vi "Reactor Coolant Pump Motor Speed.vi"(0 "SI600.lvclass in":refnum<class "SI600.lvclass">, 1 "3 JEB CS951 XQ01":dbl, 2 "3 JEB CS952 XQ01":dbl, 3 "3 JEB CS953 XQ01":dbl, 4 "3 JEB CS954 XQ01":dbl, 5 "error in":errorcluster) -> (14 "SI600.lvclass out":refnum<class "SI600.lvclass">, 15 "RCP20 Speed":dbl, 16 "Speed Calculations":T2, 17 "Speed per Loop":T1, 19 "error IO":errorcluster)   [LabVIEW 2022 SP3, in "SI600.lvclass"]
uses:
  SI600.lvclass
  SI600.lvclass/SI600.ctl
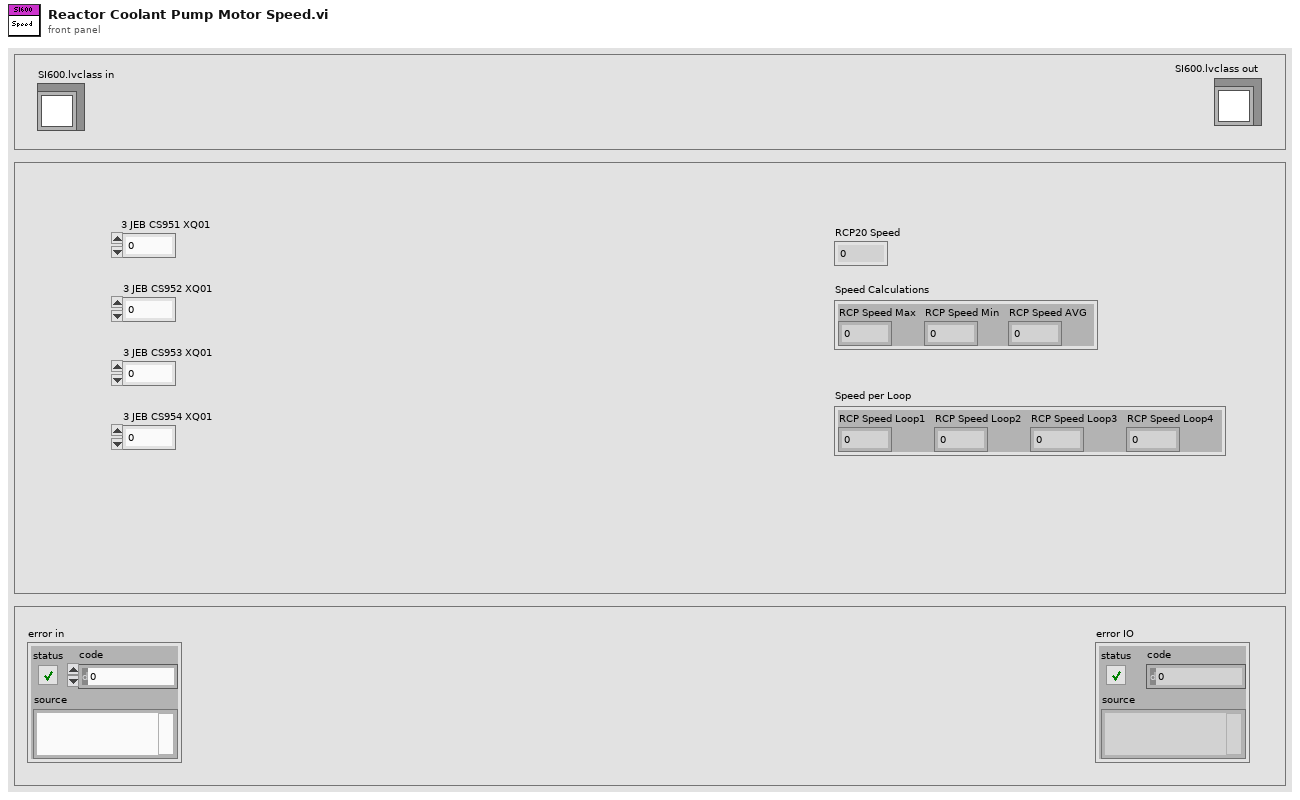
[diagram p1: front panel]
types:
  T1 = cluster{"RCP Speed Loop1":dbl, "RCP Speed Loop2":dbl, "RCP Speed Loop3":dbl, "RCP Speed Loop4":dbl}
  T2 = cluster{"RCP Speed Max":dbl, "RCP Speed Min":dbl, "RCP Speed AVG":dbl}
  T3 = cluster{"3 JEB CS951 ":dbl, "3 JEB CS952":dbl, "3 JEB CS953":dbl, "3 JEB CS954":dbl}
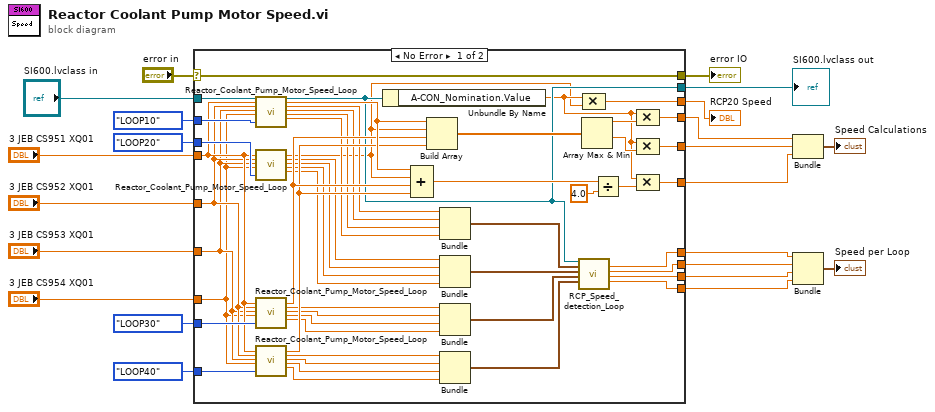
[diagram p0: block diagram]
diagram:
  n1 = case shown="No Error" "error in" {
    selector: "error in" -> [w27 w73]
    tunnel: enum16{"LOOP10", "LOOP20", "LOOP30", "LOOP40"}."LOOP10" ("Loop") -> [w69 _]
    tunnel: enum16{"LOOP10", "LOOP20", "LOOP30", "LOOP40"}."LOOP20" ("Loop") -> [w68 _]
    tunnel: enum16{"LOOP10", "LOOP20", "LOOP30", "LOOP40"}."LOOP30" ("Loop") -> [w72 _]
    tunnel: enum16{"LOOP10", "LOOP20", "LOOP30", "LOOP40"}."LOOP40" ("Loop") -> [w71 _]
    tunnel: "SI600.lvclass in" -> [w70 w74]
    tunnel: [w37 w74] -> w16
    tunnel: [w41 _] -> w9
    tunnel: [w40 _] -> w8
    tunnel: [w39 _] -> w7
    tunnel: [w38 _] -> w6
    tunnel: [w35 _] -> w12
    tunnel: [w33 _] -> w13
    tunnel: [w31 _] -> w11
    tunnel: [w28 _] -> w15
    tunnel: [w27 w73] -> w14
    tunnel: "3 JEB CS951 XQ01" -> [w26 _]
    tunnel: "3 JEB CS952 XQ01" -> [w25 _]
    tunnel: "3 JEB CS953 XQ01" -> [w24 _]
    tunnel: "3 JEB CS954 XQ01" -> [w23 _]
    frame No Error {
      n2 = call "Reactor_Coolant_Pump_Motor_Speed_Loop.vi"("SI600.lvclass in"=w70, "3 JEB CS951 XQ01"=w26, "3 JEB CS952 XQ01"=w25, "3 JEB CS953 XQ01"=w24, "3 JEB CS954 XQ01"=w23, "Loop"=w69) -> ("SI600.lvclass out"=w37:refnum<class "SI600.lvclass">, "RCP speed Loop Output"=w66:dbl, "3 JEB CS951"=w61:dbl, "3 JEB CS952"=w60:dbl, "3 JEB CS953"=w59:dbl, "3 JEB CS954"=w58:dbl)  [unwired: 15 in, 1 out]
      n3 = call "Reactor_Coolant_Pump_Motor_Speed_Loop.vi"("3 JEB CS951 XQ01"=w26, "3 JEB CS952 XQ01"=w25, "3 JEB CS953 XQ01"=w24, "3 JEB CS954 XQ01"=w23, "Loop"=w68) -> ("RCP speed Loop Output"=w29:dbl, "3 JEB CS951"=w56:dbl, "3 JEB CS952"=w55:dbl, "3 JEB CS953"=w54:dbl, "3 JEB CS954"=w53:dbl)  [unwired: 16 in, 2 out]
      n4 = call "Reactor_Coolant_Pump_Motor_Speed_Loop.vi"("3 JEB CS951 XQ01"=w26, "3 JEB CS952 XQ01"=w25, "3 JEB CS953 XQ01"=w24, "3 JEB CS954 XQ01"=w23, "Loop"=w72) -> ("RCP speed Loop Output"=w65:dbl, "3 JEB CS951"=w51:dbl, "3 JEB CS952"=w50:dbl, "3 JEB CS953"=w49:dbl, "3 JEB CS954"=w48:dbl)  [unwired: 16 in, 2 out]
      n5 = call "Reactor_Coolant_Pump_Motor_Speed_Loop.vi"("3 JEB CS951 XQ01"=w26, "3 JEB CS952 XQ01"=w25, "3 JEB CS953 XQ01"=w24, "3 JEB CS954 XQ01"=w23, "Loop"=w71) -> ("RCP speed Loop Output"=w64:dbl, "3 JEB CS951"=w46:dbl, "3 JEB CS952"=w45:dbl, "3 JEB CS953"=w44:dbl, "3 JEB CS954"=w43:dbl)  [unwired: 16 in, 2 out]
      n6 = Unbundle By Name(w37) -> ("A-CON_Nomination.Value"=w30:dbl)
      n7 = Compound Arithmetic op=ADD(w66, w29, w65, w64) -> (w63:dbl)
      n8 = Build Array(w66, w29, w65, w64) -> (w67:dbl[])
      n9 = Bundle("3 JEB CS951"=w61, "3 JEB CS952"=w60, "3 JEB CS953"=w59, "3 JEB CS954"=w58) -> (w57:T3)  [unwired: 1 in]
      n10 = Bundle("3 JEB CS951"=w56, "3 JEB CS952"=w55, "3 JEB CS953"=w54, "3 JEB CS954"=w53) -> (w52:T3)  [unwired: 1 in]
      n11 = Bundle("3 JEB CS951"=w51, "3 JEB CS952"=w50, "3 JEB CS953"=w49, "3 JEB CS954"=w48) -> (w47:T3)  [unwired: 1 in]
      n12 = Bundle("3 JEB CS951"=w46, "3 JEB CS952"=w45, "3 JEB CS953"=w44, "3 JEB CS954"=w43) -> (w42:T3)  [unwired: 1 in]
      n13 = call "RCP_Speed_detection_Loop.vi"("SI600.lvclass"=w37, "Loop10"=w57, "Loop20"=w52, "Loop30"=w47, "Loop40"=w42) -> ("RCP Speed Loop1"=w41:dbl, "RCP Speed Loop2"=w40:dbl, "RCP Speed Loop3"=w39:dbl, "RCP Speed Loop4"=w38:dbl)  [unwired: 9 in, 2 out]
      n14 = Array Max & Min(array=w67) -> (max value=w34:dbl, min value=w36:dbl)  [unwired: 2 out]
      n15 = Compound Arithmetic op=MULTIPLY(w30, w29) -> (w28:dbl)
      n16 = Divide(x=w63, y=4.0) -> (x/y=w32:dbl)
      n17 = Compound Arithmetic op=MULTIPLY(w30, w34) -> (w33:dbl)
      n18 = Compound Arithmetic op=MULTIPLY(w30, w36) -> (w35:dbl)
      n19 = Compound Arithmetic op=MULTIPLY(w30, w32) -> (w31:dbl)
    }
    frame Error {
    }
  }
  "SI600.lvclass out" <- w16
  "RCP20 Speed" <- w15
  "error IO" <- w14
  n20 = Bundle(w13, w12, w11) -> (→"Speed Calculations":cluster{dbl, dbl, dbl})  [unwired: 1 in]
  n21 = Bundle("RCP Speed Loop1"=w9, "RCP Speed Loop2"=w8, "RCP Speed Loop3"=w7, "RCP Speed Loop4"=w6) -> (→"Speed per Loop":T1)  [unwired: 1 in]
